vi "Send.vi"(8 "Error In":errorcluster, 10 "Message":string, 11 "reference in":refnum<class "Colleague.lvclass">) -> (0 "Error Out":errorcluster, 3 "reference out":refnum<class "Colleague.lvclass">)   [LabVIEW 2020, in "Colleague.lvclass"]
uses:
  Colleague.lvclass
  Mediator_class/Mediator.lvclass
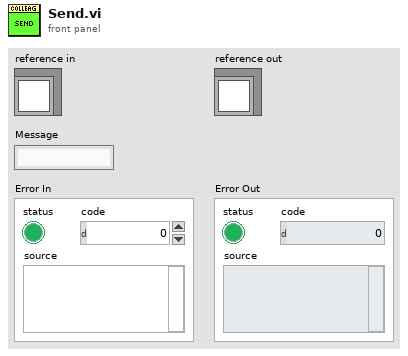
[diagram p1: front panel]
types:
  T1 = typedef "Colleague.lvclass/ObjectAttributes.ctl" = cluster{"Mediator":refnum<class "Mediator.lvclass">}
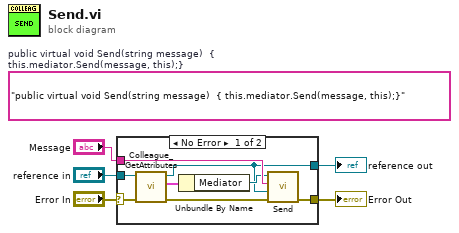
[diagram p0: block diagram]
diagram:
  (unwired) "public virtual void Send(string message)  { this.mediator.Send(message, this);}"  # public virtual void Send(string message)  { this.mediator.Send(message, this);}
  n1 = case shown="No Error" "Error In" {
    selector: "Error In" -> [w12 w15]
    tunnel: [w7 w15] -> w4
    tunnel: [w6 w14] -> w2
    tunnel: "reference in" -> [w13 w14]
    tunnel: "Message" -> [w11 _]
    frame No Error {
      n2 = call "Colleague_GetAttributes.vi"("error in (no error)"=w12, "reference in"=w13) -> ("error out"=w8:errorcluster, "Data"=w9:T1, "reference out"=w6:refnum<class "Colleague.lvclass">)  [unwired: 6 in, 1 out]
      n3 = Unbundle By Name(w9) -> ("Mediator"=w10:refnum<class "Mediator.lvclass">)
      n4 = call-dynamic "Send.vi"("Error In"=w8, "Colleague"=w6, "Message"=w11, "reference in"=w10) -> ("Error Out"=w7:errorcluster)  [unwired: 6 in, 1 out]
    }
    frame Error {
    }
  }
  "Error Out" <- w4
  "reference out" <- w2
